vi "Initialize Attributes.vi"(8 "error in (no error)":errorcluster, 10 "Attribute Data":variant, 11 "CS++DSCMsgLogger in":refnum<class "CS++DSCMsgLogger.lvclass">) -> (0 "error out":errorcluster, 2 "Found?":bool, 3 "CS++DSCMsgLogger out":refnum<class "CS++DSCMsgLogger.lvclass">)   [LabVIEW 2015, in "CS++DSCMsgLogger.lvlib" / "CS++DSCMsgLogger.lvclass"]
doc: "Initialize object attribute.\n\nUnique resources should be allocated elsewhere!"
uses:
  CS++DSCMsgLogger.lvclass
  CS++DSCMsgLogger.lvclass/CS++DSCMsgLogger.ctl
  CSPP_Core/Classes/CS++BaseClasses/MessageLogger/CS++MessageLogger.lvclass
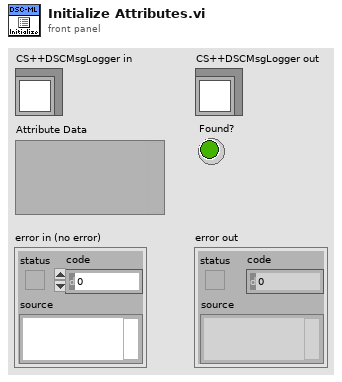
[diagram p1: front panel]
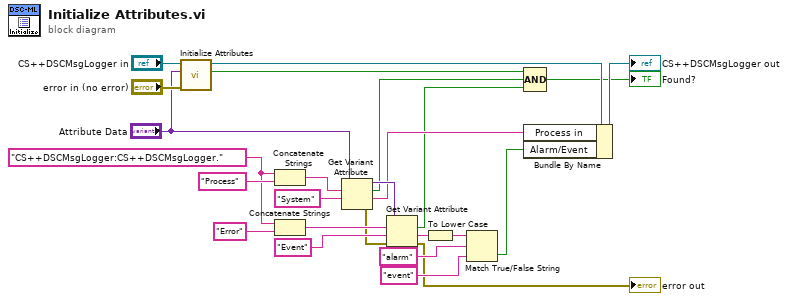
[diagram p0: block diagram]
diagram:
  w13 = "CS++DSCMsgLogger:CS++DSCMsgLogger." ("name")
  n1 = call-parent "Initialize Attributes.vi"("error in (no error)"="error in (no error)", "Attribute Data"="Attribute Data", "CS++Base in"="CS++DSCMsgLogger in") -> ("Found?"=w2:bool, "CS++Base out"=w8:refnum<class "CS++DSCMsgLogger.lvclass">)  [unwired: 6 in, 1 out]
  n2 = Concatenate Strings(w13, "Process" ("name")) -> (w14:string)
  n3 = Concatenate Strings(w13, "Error" ("name")) -> (w11:string)
  n4 = Get Variant Attribute(Variant="Attribute Data", name=w14, default value (empty Variant)="System" ("name")) -> (duplicate Variant=w22:variant, found=w4:bool, value=w6:string, error out=w10:errorcluster)  [unwired: 1 in]
  n5 = Get Variant Attribute(Variant=w22, name=w11, default value (empty Variant)="Event" ("name"), error in=w10) -> (found=w3:bool, value=w21:string, error out=→"error out":errorcluster)  [unwired: 1 out]
  n6 = To Lower Case(string=w21) -> (all lower case string=w20:string)
  n7 = Match True/False String(2:"event" ("false string"), 3:"alarm" ("string"), 4:w20) -> (0:w5:bool)  [unwired: 1 out]
  n8 = Compound Arithmetic op=AND(w2, w4, w3) -> (→"Found?":bool)
  n9 = Bundle By Name(cluster=w8, "Process in"=w6, "Alarm/Event"=w5) -> (→"CS++DSCMsgLogger out":refnum<class "CS++DSCMsgLogger.lvclass">)
